vi "功能试验 扭矩最值.vi"(9 "扭矩正转2":dbl[](array[numeric]), 10 "扭矩反转":dbl[](array[numeric]), 11 "扭矩正转1":dbl[](array[numeric])) -> (0 "反转最小值":dbl, 1 "反转最大值":dbl, 2 "正转最小值":dbl, 3 "正转最大值":dbl)   [LabVIEW 2015, in "Logging.lvlib"]
uses:
  Logging.lvlib
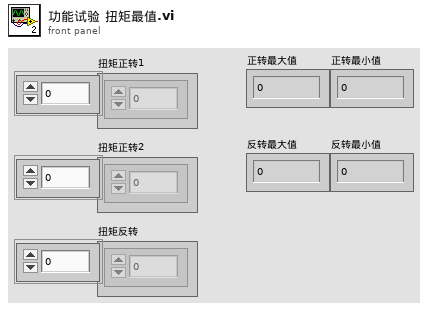
[diagram p1: front panel]
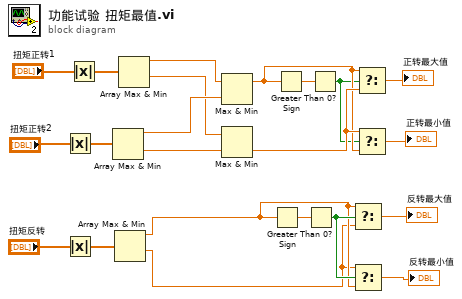
[diagram p0: block diagram]
diagram:
  n1 = Absolute Value(x="扭矩正转2") -> (abs(x)=w3:dbl[])
  n2 = Absolute Value(x="扭矩反转") -> (abs(x)=w5:dbl[])
  n3 = Absolute Value(x="扭矩正转1") -> (abs(x)=w1:dbl[])
  n4 = Array Max & Min(array=w3) -> (max value=w21:dbl, min value=w18:dbl)  [unwired: 2 out]
  n5 = Array Max & Min(array=w5) -> (max value=w10:dbl, min value=w9:dbl)  [unwired: 2 out]
  n6 = Array Max & Min(array=w1) -> (max value=w22:dbl, min value=w19:dbl)  [unwired: 2 out]
  n7 = Max & Min(x=w22, y=w21) -> (max(x,y)=w15:dbl)  [unwired: 1 out]
  n8 = Max & Min(x=w19, y=w18) -> (min(x,y)=w16:dbl)  [unwired: 1 out]
  n9 = Sign(1:w10) -> (0:w12:dbl)
  n10 = Sign(1:w15) -> (0:w20:dbl)
  n11 = Greater Than 0?(x=w12) -> (x > 0?=w11:bool)
  n12 = Greater Than 0?(x=w20) -> (x > 0?=w14:bool)
  n13 = Select(t=w10, s=w11, f=w9) -> (s? t:f=→"反转最大值":dbl)
  n14 = Select(t=w9, s=w11, f=w10) -> (s? t:f=→"反转最小值":dbl)
  n15 = Select(t=w15, s=w14, f=w16) -> (s? t:f=→"正转最大值":dbl)
  n16 = Select(t=w16, s=w14, f=w15) -> (s? t:f=→"正转最小值":dbl)
